vi "productsLow.vi"(8 "error in (no error)":errorcluster, 11 "reference in":refnum<class "Project Panels.lvclass">=refnum) -> (0 "error out":errorcluster, 3 "reference out":refnum<class "Project Panels.lvclass">)   [LabVIEW 2015, in "Project Panels.lvclass"]
uses:
  Project Panels.lvclass
  state.ctl
  <vilib>/Utility/miscctls.llb/LVRowAndColumnUnsignedTypeDef.ctl
  SYS/Devices Controller_llb/deviceType.ctl
  <vilib>/Utility/miscctls.llb/LVRowAndColumnTypeDef.ctl
  SYS/Devices Controller_llb/Devices Controller.lvclass
panel:
  out "title":string="Cosmed Asia Pacific - Products in Aussie"
  in  "tables":T1(tab)
  out "K5":string[][](table)=[["705001", "not active", "K4b2", "not active", "not active", "not active", "not active", "not active", "not active", "not active", "not active", "not active", ""], ["803033", "not active", "K4b2", "not active", "not active", "not active", "not active", "not active", "not active", "not active", "not active", "not active", ""], ["804042", "not active", "K4b2", "not active", "not active", "not active", "not active", "not active", "not active", "not active", "not active", "not active", ""], ["804046", "", "K4b2", "Univ. of Queensland", "St Lucia, Brisbane", "Gary Wilson", "seant@hms.uq.edu.au", "Bellamby", "sep-06", "Italy", "sep-07", "not active", ""], ["804047", "not active", "K4b2", "not active", "not active", "not active", "not active", "not active", "not active", "not active", "not active", "not active", ""], ["9806059", "6.2", "K4b2", "not active", "not active", "not active", "not active", "not active", "not active", "not active", "not active", "not active", ""], ["9806062", "5.1", "K4b2", "Queensland Academy of Sport", "Sunnybank", "Mark Andrews", "mark.andrews@srq.qld.com.au", "Nahtan, GC", "june 2013 in italy for CO2 refurbish", "Italy service", "jun-14", "", ""], ["9807077", "6.0a", "K4b2", "Uni of Canterbury", "Uni of Canterbury", "Gavin Blackwell", "gavin.blackwell@canterbury.ac.nz", "Christchurch", "feb-13", "fede", "feb-14", "", ""], ["9810080", "", "K4b2", "Royal Children's Hospital", "Herston", "Teresa Phillips", "Teresa_Phillips@health.qld.gov.au", "Herston", "jun-06", "Italy", "jun-07", "9/17/2013", ""], ["9903123", "7.2", "K4b2", "Uni of Adelaide", "Uni of Adelaide", "David Bentley", "david.bentley@adelaide.edu.au", "Adelaide", "dic-12", "Serv Italy +valve", "dic-13", "", ""], ["9912206", "7.3", "K4b2", "Uni of Canterbury", "Uni of Canterbury", "Gavin Blackwell", "gavin.blackwell@canterbury.ac.nz", "Christchurch", "feb-13", "fede", "feb-14", "", ""], ["200104325", "8", "K4b2", "Uni of South Australia", "Sansom Institute", "Michelle N. McDonnell", "", "Adelaide", "nov-11", "fede", "dic-12", "9/9/2013", ""], ["200201385", "9.1b", "K4b2", "University of Sydney", "Lidcombe Campus", "Hui Yin Ler  (PhD)", "", "Sydney", "oct-11", "fede", "oct-12", "9/9/2013", ""], ["200205419", "8.0", "K4b2", "University of Sydney", "Liverpool hospital", "Leanne Hassett", "leanne.hassett@sydney.edu.au", "Sydney", "nov-11", "fede", "nov-12", "Not Using in this moment", ""], ["200205423", "9.1b", "K4b2", "University of Sydney", "Lidcombe Campus", "Martin Thomson", "", "Sydney", "feb-10", "italy", "feb-11", "9/9/2013", ""], ["200205424", "7.3", "K4b2", "University of Sydney", "Lidcombe Campus", "Martin Thomson", "", "Sydney", "sep-08", "Italy", "sep-09", "9/10/2013", ""], ["200404607", "", "K4b2", "The Sydney Children's Hospital Network", "Westmead", "Leanne Purcell", "leanne.purcell@health.nsw.gov.au", "Westmead", "nov-08", "italy", "nov-09", "9/17/2013", "Yes, but waiting the start of the testing"], ["200512701", "8.0b", "K4b2", "James Cook Uni", "James Cook Uni", "Anthony Leight", "Anthony.Leicht@jcu.edu.au", "Townsville", "jan-13", "", "jan-14", "", ""], ["200601705", "", "K4b2", "Latrobe University", "Bundoora (Melb)", "Paul Moon", "P.Moon@latrobe.edu.au", "Melbourne", "jan-08", "Italy", "jan-09", "9/17/2013", ""], ["200607745", "", "K4b2", "QUT Brisbane", "Kelvin Grove", "Pei Cher", "pei.cher@qut.edu.au", "BBN", "may-13", "fede", "may-14", "", ""], ["200710813", "", "K4b2", "Victoria Uni", "", "Jessica Meilak", "jessica.meilak@vu.edu.au", "Melb", "jan-12", "Brad", "jan-14", "15/01/14", ""], ["200907909", "9.1b", "K4b2", "Uni of New South Wales", "Uni of New South Wales", "Stephen Redmond", "s.redmond@unsw.edu.au", "Sydney", "sep-12", "fede", "sep-13", "9/17/2013", ""], ["200909916", "", "K4b2", "Uni of Canterbury", "Uni of Canterbury", "Gavin Blackwell", "gavin.blackwell@canterbury.ac.nz", "Christchurch", "feb-13", "fede", "feb-14", "", ""], ["201007964", "", "K4b2", "University of Canberra", "Canberra", "Ben Rattray", "ben.rattray@canberra.edu.au", "Canberra", "mar-12", "", "mar-13", "9/17/2013", ""], ["201009980", "9.1b", "K4b2", "Uni of Technology Sydney", "UTS City Campus", "Steven Su", "steven.su@eng.uts.edu.au", "Sydney", "oct-12", "Medtel (also Lee Valve)", "oct-13", "9/17/2013", ""], ["2011121063", "", "K4b2", "Victoria Uni", "", "Jessica Meilak", "jessica.meilak@vu.edu.au", "Melb", "jan-12", "Brad", "jan-14", "", ""], ["2011121064", "", "K4b2", "Victoria Uni", "", "Jessica Meilak", "jessica.meilak@vu.edu.au", "Melb", "jan-12", "Brad", "jan-14", "", ""], ["2012021076", "", "K4b2", "Demo Unit", "Demo Unit", "TBD", "", "TBD", "sep-13", "Manu-AUS", "sep-14", "", ""], ["2012021080", "", "K4b2", "Massey Univ.", "Wellington", "Brandon Woolley", "B.Woolley@massey.ac.nz", "Wellington", "nov-13", "Manu-AUS", "nov-14", "", ""], ["2012061109", "", "K4b2", "Griffith University Gold Coast Campus", "Gold Coast", "Anna Boehm", "a.boehm@griffith.edu.au", "Gold Coast", "jul-13", "fede", "jul-14", "", ""], ["2012061115", "10.0d", "K4b2", "University of Newcastle", "Callaghan", "Robin Callister", "Robin.Callister@newcastle.edu.au", "Ourimbah", "nov-13", "Manu-AUS", "nov-14", "", ""], ["2012111144", "10.0d", "K4b2", "University of Newcastle", "Callaghan", "Robin Callister", "Robin.Callister@newcastle.edu.au", "Ourimbah", "nov-13", "Manu-AUS", "nov-14", "", ""], ["2012111148", "", "K4b2", "University of Western Sydney", "PENRITH", "Tara Hamilton", "t.hamilton@uws.edu.au", "PENRITH", "dec-13", "Manu-AUS", "dec-14", "", ""], ["2013011158", "10.0d", "K4b2", "University of the Sunshine Coast", "Maroochydore DC", "Ava Kerr", "akerr@usc.edu.au", "Sippy Downs", "may-13", "new", "may-14", "", ""], ["2013031168", "10.0d", "K4b2", "Australian Catholic University", "Sydney", "Phillip Chapman", "Phillip.Chapman@acu.edu.au", "Sydney", "apr-13", "new", "apr-14", "", ""], ["Prova", "", "Prova", "", "", "", "", "", "", "", "", "", ""]]
  out "k4b2":string[][](table)=[["705001", "not active", "K4b2", "not active", "not active", "not active", "not active", "not active", "not active", "not active", "not active", "not active", ""], ["803033", "not active", "K4b2", "not active", "not active", "not active", "not active", "not active", "not active", "not active", "not active", "not active", ""], ["804042", "not active", "K4b2", "not active", "not active", "not active", "not active", "not active", "not active", "not active", "not active", "not active", ""], ["804046", "", "K4b2", "Univ. of Queensland", "St Lucia, Brisbane", "Gary Wilson", "seant@hms.uq.edu.au", "Bellamby", "sep-06", "Italy", "sep-07", "not active", ""], ["804047", "not active", "K4b2", "not active", "not active", "not active", "not active", "not active", "not active", "not active", "not active", "not active", ""], ["9806059", "6.2", "K4b2", "not active", "not active", "not active", "not active", "not active", "not active", "not active", "not active", "not active", ""], ["9806062", "5.1", "K4b2", "Queensland Academy of Sport", "Sunnybank", "Mark Andrews", "mark.andrews@srq.qld.com.au", "Nahtan, GC", "june 2013 in italy for CO2 refurbish", "Italy service", "jun-14", "", ""], ["9807077", "6.0a", "K4b2", "Uni of Canterbury", "Uni of Canterbury", "Gavin Blackwell", "gavin.blackwell@canterbury.ac.nz", "Christchurch", "feb-13", "fede", "feb-14", "", ""], ["9810080", "", "K4b2", "Royal Children's Hospital", "Herston", "Teresa Phillips", "Teresa_Phillips@health.qld.gov.au", "Herston", "jun-06", "Italy", "jun-07", "9/17/2013", ""], ["9903123", "7.2", "K4b2", "Uni of Adelaide", "Uni of Adelaide", "David Bentley", "david.bentley@adelaide.edu.au", "Adelaide", "dic-12", "Serv Italy +valve", "dic-13", "", ""], ["9912206", "7.3", "K4b2", "Uni of Canterbury", "Uni of Canterbury", "Gavin Blackwell", "gavin.blackwell@canterbury.ac.nz", "Christchurch", "feb-13", "fede", "feb-14", "", ""], ["200104325", "8", "K4b2", "Uni of South Australia", "Sansom Institute", "Michelle N. McDonnell", "", "Adelaide", "nov-11", "fede", "dic-12", "9/9/2013", ""], ["200201385", "9.1b", "K4b2", "University of Sydney", "Lidcombe Campus", "Hui Yin Ler  (PhD)", "", "Sydney", "oct-11", "fede", "oct-12", "9/9/2013", ""], ["200205419", "8.0", "K4b2", "University of Sydney", "Liverpool hospital", "Leanne Hassett", "leanne.hassett@sydney.edu.au", "Sydney", "nov-11", "fede", "nov-12", "Not Using in this moment", ""], ["200205423", "9.1b", "K4b2", "University of Sydney", "Lidcombe Campus", "Martin Thomson", "", "Sydney", "feb-10", "italy", "feb-11", "9/9/2013", ""], ["200205424", "7.3", "K4b2", "University of Sydney", "Lidcombe Campus", "Martin Thomson", "", "Sydney", "sep-08", "Italy", "sep-09", "9/10/2013", ""], ["200404607", "", "K4b2", "The Sydney Children's Hospital Network", "Westmead", "Leanne Purcell", "leanne.purcell@health.nsw.gov.au", "Westmead", "nov-08", "italy", "nov-09", "9/17/2013", "Yes, but waiting the start of the testing"], ["200512701", "8.0b", "K4b2", "James Cook Uni", "James Cook Uni", "Anthony Leight", "Anthony.Leicht@jcu.edu.au", "Townsville", "jan-13", "", "jan-14", "", ""], ["200601705", "", "K4b2", "Latrobe University", "Bundoora (Melb)", "Paul Moon", "P.Moon@latrobe.edu.au", "Melbourne", "jan-08", "Italy", "jan-09", "9/17/2013", ""], ["200607745", "", "K4b2", "QUT Brisbane", "Kelvin Grove", "Pei Cher", "pei.cher@qut.edu.au", "BBN", "may-13", "fede", "may-14", "", ""], ["200710813", "", "K4b2", "Victoria Uni", "", "Jessica Meilak", "jessica.meilak@vu.edu.au", "Melb", "jan-12", "Brad", "jan-14", "15/01/14", ""], ["200907909", "9.1b", "K4b2", "Uni of New South Wales", "Uni of New South Wales", "Stephen Redmond", "s.redmond@unsw.edu.au", "Sydney", "sep-12", "fede", "sep-13", "9/17/2013", ""], ["200909916", "", "K4b2", "Uni of Canterbury", "Uni of Canterbury", "Gavin Blackwell", "gavin.blackwell@canterbury.ac.nz", "Christchurch", "feb-13", "fede", "feb-14", "", ""], ["201007964", "", "K4b2", "University of Canberra", "Canberra", "Ben Rattray", "ben.rattray@canberra.edu.au", "Canberra", "mar-12", "", "mar-13", "9/17/2013", ""], ["201009980", "9.1b", "K4b2", "Uni of Technology Sydney", "UTS City Campus", "Steven Su", "steven.su@eng.uts.edu.au", "Sydney", "oct-12", "Medtel (also Lee Valve)", "oct-13", "9/17/2013", ""], ["2011121063", "", "K4b2", "Victoria Uni", "", "Jessica Meilak", "jessica.meilak@vu.edu.au", "Melb", "jan-12", "Brad", "jan-14", "", ""], ["2011121064", "", "K4b2", "Victoria Uni", "", "Jessica Meilak", "jessica.meilak@vu.edu.au", "Melb", "jan-12", "Brad", "jan-14", "", ""], ["2012021076", "", "K4b2", "Demo Unit", "Demo Unit", "TBD", "", "TBD", "sep-13", "Manu-AUS", "sep-14", "", ""], ["2012021080", "", "K4b2", "Massey Univ.", "Wellington", "Brandon Woolley", "B.Woolley@massey.ac.nz", "Wellington", "nov-13", "Manu-AUS", "nov-14", "", ""], ["2012061109", "", "K4b2", "Griffith University Gold Coast Campus", "Gold Coast", "Anna Boehm", "a.boehm@griffith.edu.au", "Gold Coast", "jul-13", "fede", "jul-14", "", ""], ["2012061115", "10.0d", "K4b2", "University of Newcastle", "Callaghan", "Robin Callister", "Robin.Callister@newcastle.edu.au", "Ourimbah", "nov-13", "Manu-AUS", "nov-14", "", ""], ["2012111144", "10.0d", "K4b2", "University of Newcastle", "Callaghan", "Robin Callister", "Robin.Callister@newcastle.edu.au", "Ourimbah", "nov-13", "Manu-AUS", "nov-14", "", ""], ["2012111148", "", "K4b2", "University of Western Sydney", "PENRITH", "Tara Hamilton", "t.hamilton@uws.edu.au", "PENRITH", "dec-13", "Manu-AUS", "dec-14", "", ""], ["2013011158", "10.0d", "K4b2", "University of the Sunshine Coast", "Maroochydore DC", "Ava Kerr", "akerr@usc.edu.au", "Sippy Downs", "may-13", "new", "may-14", "", ""], ["2013031168", "10.0d", "K4b2", "Australian Catholic University", "Sydney", "Phillip Chapman", "Phillip.Chapman@acu.edu.au", "Sydney", "apr-13", "new", "apr-14", "", ""], ["Prova", "", "Prova", "", "", "", "", "", "", "", "", "", ""]]
  out "fitmate":string[][](table)=[["2005090013", "2.2", "Fitmate Pro", "Wesley Weight Management", "Milton", "Liz Ernst", "eernst@lifeshape.com.au", "Milton", "27/09", ""], ["2006020058", "1", "Fitmate WM", "Toombul Medical Centre", "Spring Hill", "Zoe Glover", "toombulmc@gmail.com", "Spring Hill", "27/09", ""], ["2006020059", "1", "Fitmate WM", "RMIT Univ.", "Melbourne", "George Lenon", "george.lenon@rmit.edu.au", "Melbourne", "27/09", ""], ["2006020060", "1", "Fitmate WM", "Logan Hospital", "Meadowbrook", "??", "??", "Meadowbrook", "", ""], ["2006020061", "1.6", "Fitmate WM", "Biomedex (Aust) Pty Ltd", "Woonona", "Biomedex (Aust) Pty Ltd", "??", "Woonona", "", ""], ["2006020077", "1", "Fitmate Pro", "Wesley Weight Management", "Southport", "Sally Jordan", "SJordan@weshealth.com.au", "Southport", "27/09 mail come back / no problem", ""], ["2006020078", "1", "Fitmate Pro", "Life4Ever Pty Ltd", "Arundel", "Michael Tait", "mail@drmichaeltait.com", "Arundel", "27/09 mail come back", ""], ["2006030062", "2.2", "Fitmate WM", "Biomedex (Aust) Pty Ltd", "Woonona", "Biomedex (Aust) Pty Ltd", "??", "Woonona", "", ""], ["2006030083", "2", "Fitmate Pro", "Australian College of Physical Education", "Olympic Park Sydney", "Sven Rees", "srees@acpe.edu.au", "Olympic Park Sydney", "30/09", ""], ["2006030084", "2.3", "Fitmate Pro", "Monash Univ. The Alfred Centre", "Frankston", "Tim Wallace", "tim.wallace@monash.edu", "Frankston", "Case Opned for Macro error", ""], ["2006030085", "2.2", "Fitmate Pro", "Southside Exercise Therapy", "Gymea", "Luke Delvecchio", "southsidepty@optusnet.com.au", "Gymea", "30/09", ""], ["2006060076", "1.1", "Fitmate WM", "Edith Cowan Univ.", "Joondalup", "Amanda Devine", "a.devine@ecu.edu.au", "Joondalup", "30/09", ""], ["2006060078", "1.1", "Fitmate WM", "Edith Cowan Univ.", "Joondalup", "Amanda Devine", "a.devine@ecu.edu.au", "Joondalup", "30/09", ""], ["2006060080", "2.3", "Fitmate WM", "WESLEY Corporate Health", "Brisbane", "Liz Ernst", "eernst@lifeshape.com.au", "Brisbane", "27/09", ""], ["2006080185", "1.1", "Fitmate Pro", "Edith Cowan Univ.", "Joondalup", "Doreen Mackie", "DMackie@hotmail.com", "Joondalup", "Waiting for details from email (n.vrdoljak@ecu.edu.au   )", ""], ["2006080186", "1.1", "Fitmate Pro", "Neocardia PTY LTD", "Noosaville", "Neavison", "Neavison@hotmail.com", "Noosaville", "30/09", ""], ["2006080187", "1.1", "Fitmate Pro", "Kams Health and Fitness", "Armidale", "Kamahl Barhoush", "info@kams.com.au", "Armidale", "doesn't answer/call again", ""], ["2006080188", "1.1", "Fitmate Pro", "Edith Cowan Univ.", "Joondalup", "Doreen Mackie", "DMackie@hotmail.com", "Joondalup", "Waiting for details from email (n.vrdoljak@ecu.edu.au   )", ""], ["2006080189", "1.1", "Fitmate Pro", "Get Back On Track", "Victoria", "Lisa Ham", "LisaH@bigpond.com.au", "Victoria", "doesn't answer/call again", ""], ["2006080190", "1.1", "Fitmate Pro", "Edith Cowan Univ.", "Joondalup", "Doreen Mackie", "DMackie@hotmail.com", "Joondalup", "Waiting for details from email (n.vrdoljak@ecu.edu.au   )", ""], ["2006080191", "1.1", "Fitmate Pro", "One Life", "PADDINGTON", "Justin Lang", "admin@onelifeliveit.net.au", "PADDINGTON", "01/10", "NOT ACTIVE"], ["2007030363", "1.1", "Fitmate Pro", "X-Fitness Systems Ltd", "Auckland,", "Scott Tibbutt", "scott@xfitness.co.nz", "Auckland,", "30/09", ""], ["2007030372", "1.1", "Fitmate Pro", "Edith Cowan Univ.", "Joondalup", "Doreen Mackie", "DMackie@hotmail.com", "Joondalup", "Waiting for details from email (n.vrdoljak@ecu.edu.au   )", ""], ["2007030373", "1.1", "Fitmate Pro", "Edith Cowan Univ.", "Joondalup", "Doreen Mackie", "DMackie@hotmail.com", "Joondalup", "Waiting for details from email (n.vrdoljak@ecu.edu.au   )", ""], ["2007030375", "1.1", "Fitmate Pro", "Vision Health and Fitness", "Toowoomba", "Troy Taylor", "troy@visionhealth.com.au", "Toowoomba", "30/09", ""], ["2007050155", "2", "Fitmate WM", "Fitness Fusion", "Ohope", "Erin Baker", "paul@fitnessfusion.co.nz", "Ohope", "30/09", ""], ["2007050156", "1.1", "Fitmate WM", "X-Fitness Systems Ltd", "Auckland,", "X-Fitness Systems Ltd", "jeremyu@uhl.co.nz", "Auckland,", "30/09", ""], ["2007050157", "2.2", "Fitmate WM", "Wesley Weight Management", "Milton", "Liz Ernst", "eernst@lifeshape.com.au", "Milton", "27/09", ""], ["2007050158", "2.2", "Fitmate WM", "WESLEY Corporate Health", "Brisbane", "Liz Ernst", "eernst@lifeshape.com.au", "Brisbane", "27/09", ""], ["2007050159", "1.1", "Fitmate WM", "Wesley Weight Management", "Rockhampton", "Simon Fawssett", "sfawssett@weshealth.com.au", "Rockhampton", "no problem", ""], ["2007050160", "2.2", "Fitmate WM", "WESLEY Corporate Health", "Brisbane", "Liz Ernst", "eernst@lifeshape.com.au", "Brisbane", "27/09", ""], ["2007050161", "1.1", "Fitmate WM", "Pyrmont Health & Fitness Club", "Pyrmont", "Antoine Poulter", "??", "Pyrmont", "", ""], ["2007050376", "1.1", "Fitmate Pro", "Edith Cowan Univ.", "Joondalup", "Doreen Mackie", "DMackie@hotmail.com", "Joondalup", "Waiting for details from email (n.vrdoljak@ecu.edu.au   )", ""], ["2007050377", "1.1", "Fitmate Pro", "Elgin Street Medical Centre", "Carlton", "Daniel Cobb", "dcobb@live.com.au", "Carlton", "30/09", ""], ["2007050378", "1.1", "Fitmate Pro", "Pyrmont Health & Fitness Club", "Pyrmont", "Justine Justine", "??", "Pyrmont", "", ""], ["2007050379", "1.6", "Fitmate Pro", "HERT", "Millers Point", "Mark Newton", "mark@hert.com.au", "Millers Point", "30/09", ""], ["2007050380", "1.1", "Fitmate Pro", "Edith Cowan Univ.", "Joondalup", "Doreen Mackie", "DMackie@hotmail.com", "Joondalup", "Waiting for details from email (n.vrdoljak@ecu.edu.au   )", ""], ["2007050381", "1.6", "Fitmate Pro", "Fitness Development Australia", "Sydney", "Fitness Development Australia", "zarko_mikulic@hotmail.com", "Sydney", "30/09", ""], ["2007050388", "1.1", "Fitmate Pro", "ULO Pty Ltd", "Roebourne Court", "Adam Brown", "adam@ulo.com.au", "Daisy Hill", "30/09", ""], ["2007050395", "1.6", "Fitmate Pro", "Biomedex (Aust) Pty Ltd", "Woonona", "Biomedex (Aust) Pty Ltd", "??", "Woonona", "", ""], ["2007050404", "1.1", "Fitmate Pro", "Biomedex (Aust) Pty Ltd", "Woonona", "Biomedex (Aust) Pty Ltd", "??", "Woonona", "", ""], ["2007060413", "2", "Fitmate Pro", "Biomedex (Aust) Pty Ltd", "Woonona", "Biomedex (Aust) Pty Ltd", "??", "Woonona", "", ""], ["2007060415", "1.1", "Fitmate Pro", "Mater Childrens Hospital", "South Brisbane", "Gary Leong", "gary.leong@mater.org.au", "South Brisbane", "1/10/2013", ""], ["2007060417", "1.1", "Fitmate Pro", "Ray Kelly Fitness", "Blacktown", "Ray Kelly", "maxvel01@hotmail.com", "Blacktown", "30/09", ""], ["2007100277", "2.2", "Fitmate WM", "Biomedex (Aust) Pty Ltd", "Woonona", "Biomedex (Aust) Pty Ltd", "??", "Woonona", "", ""], ["2007100278", "1.1", "Fitmate WM", "Tone Up Weight Loss", "Campbelltown", "Christopher Satara", "scott@swphysio.com.au'", "Campbelltown", "08/10", ""], ["2007100279", "1.6", "Fitmate WM", "Biomedex (Aust) Pty Ltd", "Woonona", "Biomedex (Aust) Pty Ltd", "??", "Woonona", "", ""], ["2007100281", "2.2", "Fitmate WM", "Biomedex (Aust) Pty Ltd", "Woonona", "Biomedex (Aust) Pty Ltd", "??", "Woonona", "", ""], ["2007100282", "2.2", "Fitmate WM", "Biomedex (Aust) Pty Ltd", "Woonona", "Biomedex (Aust) Pty Ltd", "??", "Woonona", "", ""], ["2007100484", "2.3", "Fitmate Pro", "Univ. of Auckland", "Auckland", "Grant Mawston", "", "Auckland", "", ""], ["2008010568", "2.3", "Fitmate Pro", "Australian College of", "Olympic Park Sydney", "Sven Rees", "srees@acpe.edu.au", "Olympic Park Sydney", "30/09", ""], ["2008010576", "2.2", "Fitmate Pro", "Body Dynamics Illawarra", "Bulli", "Alan Wilkie", "alan@bodydynamics.com.au", "Bulli", "01/10", ""], ["2008010578", "2.2", "Fitmate Pro", "Cardiofirst Pty Ltd.", "Frenchs Forest", "Camilla", "reports@cardiofirst.com.au", "Frenchs Forest", "", ""], ["2008010579", "2.2", "Fitmate Pro", "Biomedex (Aust) Pty Ltd", "Woonona", "Biomedex (Aust) Pty Ltd", "??", "Woonona", "", ""], ["2008010585", "1.1", "Fitmate Pro", "Biomedex (Aust) Pty Ltd", "Woonona", "Biomedex (Aust) Pty Ltd", "??", "Woonona", "", ""], ["2008030035", "1.6", "Fitmate MED", "Biomedex (Aust) Pty Ltd", "Woonona", "Biomedex (Aust) Pty Ltd", "??", "Woonona", "", ""], ["2008030037", "2", "Fitmate MED", "Biomedex (Aust) Pty Ltd", "Woonona", "Biomedex (Aust) Pty Ltd", "??", "Woonona", "", ""], ["2008040639", "1.5", "Fitmate Pro", "", "Wellington", "Stefan Darrall", "stefan.darrall@xtra.co.nz", "Wellington", "01/10", ""], ["2008040645", "2,2", "Fitmate Pro", "FEDERICO ZANELLA", "Narrabeen", "Federico Zanella", "", "Narrabeen", "", ""], ["2008090067", "2", "Fitmate MED", "Biomedex Pty Ltd.", "Bellambi", "Biomedex Pty Ltd.", "??", "Bellambi", "", ""], ["2008090071", "2", "Fitmate MED", "Logan City Council", "Logan Central", "Campbell MacGregor (not work there anymore)", "council@logan.qld.gov.au", "Logan Central", "08/10 request info sent", ""], ["2008090073", "1.6", "Fitmate MED", "Biomedex (Aust) Pty Ltd", "Woonona", "Biomedex (Aust) Pty Ltd", "??", "Woonona", "", ""], ["2008090075", "1.6", "Fitmate MED", "Enriched Health and Fizzsport Physiotherapy", "Port Macquarie", "Simon Turnball", "simon.turnbull@enrichedhealth.com.au", "Port Macquarie", "01/10", ""], ["2008090076", "2", "Fitmate MED", "Biomedex Pty Ltd.", "Bellambi", "Biomedex Pty Ltd.", "??", "Bellambi", "", ""], ["2008100402", "1.6", "Fitmate WM", "LSNDS P/L", "Mount Eliza", "Andrew Harland", "lsnds@optusenet.com.au", "Mount Eliza", "", ""], ["2008100403", "2.2", "Fitmate WM", "Monash Univ. The Alfred Centre", "Melbourne", "Emma Ridley", "emma.ridley@monash.edu", "Melbourne", "01/10", ""], ["2008100404", "1.6", "Fitmate WM", "The Prince Charles Hospital", "Brisbane", "Renee Rogers", "", "Brisbane", "", ""], ["2008100405", "2.2", "Fitmate WM", "Monash Univ. The Alfred Centre", "Melbourne", "Emma Ridley", "emma.ridley@monash.edu", "Melbourne", "01/10", ""], ["2008100408", "1.6", "Fitmate WM", "Univ. of Newcastle (AUSTRALIA)", "Tamworth", "Leanne Brown", "leanne.brown@newcastle.edu.au", "Tamworth", "01/10", ""], ["2009070009", "1,6", "Fitmate Pro", "Ray Kelly Fitness", "Blacktown", "Ray Kelly", "maxvel01@hotmail.com", "Blacktown", "30/09", ""], ["2010011057", "2", "Fitmate Pro", "Swift Sports Performance Equip", "Lismore", "Mark Fisher", "mark@spe.com.au", "Lismore", "01/10", ""], ["2010021097", "2", "Fitmate Pro", "ASCENCIA Pty. Limited", "Notting Hill", "Michael Panagopoulos", "michael@ascencia.com.au", "Notting Hill", "", ""], ["2010021098", "2", "Fitmate Pro", "Melbourne Sports & Allied Health Clinic", "Essendon North", "Simon Sostaric", "simon@msahc.com.au", "Essendon North", "01/10", ""], ["2010041123", "2", "Fitmate Pro", "Pymble Ladies College", "Pymble", "Thomas Kindred", "tkindred@pymblelc.nsw.edu.au", "Pymble", "01/10", ""], ["2010041133", "2", "Fitmate Pro", "New Zealand Institute of Sport", "Wellington", "Tony Rogers", "tony.r@nzis.co.nz", "Wellington", "info da fede", ""], ["2010091200", "2", "Fitmate Pro", "Univ. of Western Sydney", "Sydney", "Andrew Webber", "a.webber@uws.edu.au / a.boros@uws.edu.au", "Sydney", "01/10", ""], ["2010091208", "2.2", "Fitmate Pro", "AusFitness Test", "Burleigh Heads", "Daniel Mckenzie", "dan@ausfitnesstest.com", "Burleigh Heads", "01/10", ""], ["2010111079", "2", "Fitmate MED", "Xceler8", "Wagga", "Kerry Podmore", "Kerry-xceler8@bigpond.com", "Wagga", "01/10", ""], ["2010121080", "2", "Fitmate MED", "", "Toormina, Boambee", "Chris Cherry", "", "Toormina, Boambee", "", ""], ["2010121084", "2", "Fitmate MED", "Victoria University", "St.ALbans", "Christos Stathis", "christos.stathis@vu.edu.au", "St.ALbans", "01/10", ""], ["2010121085", "2", "Fitmate MED", "Victoria University", "St.ALbans", "Christos Stathis", "christos.stathis@vu.edu.au", "St.ALbans", "01/10", ""], ["2010121088", "2", "Fitmate MED", "", "Melbourne Nth.", "T. Goh", "??", "Melbourne Nth.", "", ""], ["2010121250", "2.2", "Fitmate Pro", "Otago Polytechnic", "Dunedin", "Hayden Croft", "Hayden.Croft@op.ac.nz", "Dunedin", "01/10", ""], ["2011021095", "2", "Fitmate MED", "CHM Management", "South Melbourne", "Kirsty Lerm", "klerm@chm.com.au", "South Melbourne", "01/10", ""], ["2011041238", "2.2", "Fitmate WM", "University of the Sunshine Coast", "Sippy Downs", "Gary Slater", "gslater@usc.edu.au", "Maroochydore DC", "01/10", "accepted 04/10"], ["2011061360", "2.2", "Fitmate Pro", "Sports Orthopaedic and Rehabilitation", "Sydney", "Peter McDonald", "pmcdfitness@gmail.com.au'", "Sydney", "", ""], ["2011061363", "2.2", "Fitmate Pro", "Sports Orthopaedic and Rehabilitation", "Sydney", "Peter McDonald", "pmcdfitness@gmail.com.au'", "Sydney", "", ""], ["2011071270", "2.2", "Fitmate WM", "University of Otago", "Dunedin", "Gavin Hendry", "gavin.hendry@otago.ac.nz", "Dunedin", "01/10", ""], ["2011111148", "2", "Fitmate MED", "JLM Accutek Health", "Homebush", "Lorrence(Lorenzo) Platania", "??", "Homebush", "", ""], ["2011111155", "2", "Fitmate MED", "JLM Accutek Health", "Homebush", "Lorrence(Lorenzo) Platania", "??", "Homebush", "", ""], ["2011121441", "2.2", "Fitmate Pro", "The Scots College", "Bellevue Hill", "Tenzing Tsewang", "t.tsewang@tsc.nsw.edu.au", "Bellevue Hill", "01/10", ""], ["2011121443", "2.2", "Fitmate Pro", "Sydney Sports & Exercise", "Sydney Olympic Park", "Dean McNamara", "", "Sydney Olympic Park", "", ""], ["2012031327", "2.2", "Fitmate WM", "Univ. of Adelaide", "Adelaide", "Univ. of Adelaide", "", "Adelaide", "", ""], ["2012050009", "2,3", "Fitmate GS", "Belconnen Specialist Center", "Bruce-Canberra", "Mariame Iraki", "", "Bruce-Canberra", "", ""], ["2012061551", "2.2", "Fitmate Pro", "The Scots College", "Bellevue Hill", "Tenzing Tsewang", "t.tsewang@tsc.nsw.edu.au", "Bellevue Hill", "01/10", ""], ["2012061552", "2.2", "Fitmate Pro", "The Scots College", "Bellevue Hill", "Tenzing Tsewang", "t.tsewang@tsc.nsw.edu.au", "Bellevue Hill", "01/10", ""], ["2012061554", "2.2", "Fitmate Pro", "The Scots College", "Bellevue Hill", "Tenzing Tsewang", "t.tsewang@tsc.nsw.edu.au", "Bellevue Hill", "01/10", ""], ["2012091028", "2,3", "Fitmate GS", "The University of Newcastle (AUS)", "Callaghan", "Anna Bukey", "Anna.Bukey@newcastle.edu.au", "Callaghan", "01/10", ""], ["2012101617", "2.3", "Fitmate Pro", "FEDERICO ZANELLA", "Narrabeen", "Federico Zanella", "", "Narrabeen", "", ""], ["2012101619", "2.3", "Fitmate Pro", "Adelaide Exercise Physiology (AEP)", "", "Reuben Vanderzalm", "reuben@aep.net.au", "", "01/10", ""], ["2012111654", "2.2", "Fitmate Pro", "Vascular Ultrasound Partners Pty Ltd", "Adelaide", "Jim Gotting", "emac2403@gmail.com", "Adelaide", "01/10", ""], ["2013011031", "2,3", "Fitmate GS", "FEDERICO ZANELLA", "Narrabeen", "Federico Zanella", "", "Narrabeen", "", ""], ["2013021388", "2.2", "Fitmate WM", "Monash Univ. The Alfred Centre", "Melbourne", "Emma Ridley", "emma.ridley@monash.edu", "Melbourne", "01/10", ""], ["2013041734", "2.2", "Fitmate Pro", "SA Ambulance", "Eastwood", "Adam Zerner", "adam.zerner@health.sa.gov.au", "Eastwood", "01/10", ""], ["2013061753", "2.2", "Fitmate Pro", "James Cook University", "Douglas", "Anthony Leight", "Anthony.Leicht@jcu.edu.au", "Townsville", "01/10", ""], ["20050800003", "1.6", "Fitmate Pro", "Biomedex (Aust) Pty Ltd", "Woonona", "Biomedex (Aust) Pty Ltd", "??", "Woonona", "", ""]]
  out "RMR":string[][](table)=[["2009010042", "", "RMR + ICU", "Monash Univ. The Alfred Centre", "Melbourne", "Emma Ridley", "Emma.Ridley@med.monash.edu.au", "Melbourne", "", ""], ["2010020172", "", "RMR + ICU", "Prince Charles Hospital", "Brisbane", "Vanessa King", "Vanessa_King@health.qld.gov.au", "Brisbane", "", ""], ["2010080174", "", "RMR + ICU", "Monash Univ. The Alfred Centre", "Melbourne", "Emma Ridley", "Emma.Ridley@med.monash.edu.au", "Melbourne", "", ""], ["2010110180", "", "RMR + ICU", "Monash Univ. The Alfred Centre", "Melbourne", "Emma Ridley", "Emma.Ridley@med.monash.edu.au", "Melbourne", "", ""], ["2010110181", "", "RMR + ICU", "Gold Coast Hospital and Robina", "Southport", "Alan Spencer", "alan_spencer@healthqld.gov.au", "Southport", "", ""], ["2011050212", "", "RMR + ICU", "John Hunter Hospital", "New Lambton Heights", "Justin Singleton", "justin.singleton@hnehealth.nsw.gov.au", "New Lambton Heights", "", ""], ["2011110238", "", "RMR", "Royal Prince Alfred Hospital", "Camperdown", "Joanne Heyman", "joanne.heyman@sswahs.nsw.gov.au", "Camperdown", "", ""], ["2012110294", "", "RMR", "University of the Sunshine Coast", "Maroochydore DC", "Gary Slater", "gslater@usc.edu.au", "Maroochydore DC", "", ""], ["2013020316", "", "RMR + ICU", "Royal Perth Hospital", "Perth", "Wayne Epton", "wayne.epton@health.wa.gov.au", "Perth", "", ""], ["2013050335", "", "RMR + ICU", "Gold Coast Hospital and Robina", "Southport", "Alan Spencer", "alan_spencer@healthqld.gov.au", "Southport", "", ""], ["2013050332", "", "RMR", "Auckland City Hospital", "Auckland", "Shay McGuinness", "", "Auckland", "", ""], ["2013050330", "", "RMR + ICU", "University of Queensland", "Herston", "Alexia Murphy", "alexia.murphy@uq.edu.au", "Herston", "", ""]]
  out "CPET":string[][](table)=[["9807035", "5", "Quark b2", "The Royal Melbourne Institute of Technology - RMIT", "Bundoora", "", "", "", "", ""], ["9901046", "", "Quark b2", "Biomedex", "", "", "", "", "", ""], ["9905053", "5.1a", "Quark b2", "Baker Medical Research Institute", "", "", "", "", "", ""], ["200601281", "", "Quark b2", "Ultra Thoroughbred Racing Pty. Ltb", "Green Iris", "Rod Cedaro", "rod.cedaro@gmail.com", "Rod Cedaro", "", ""], ["2007060003", "", "Quark CPET", "Liverpool Hospital", "Liverpool", "Mark Newman", "Mark.Newman@sswahs.nsw.gov.au", "Liverpool", "", ""], ["2008030037", "10.0d", "Quark CPET", "University Otago", "Dunedin", "Nigel Barrett", "nigel.barrett@otago.ac.nz", "Dunedin", "", ""], ["2008030006", "", "Quark PFT/CPET Nutritional", "University Otago", "Dunedin", "Dene Irvine", "dene.irvine@otago.ac.nz", "Dunedin", "", ""], ["2008050039", "9", "Quark CPET", "Victorian Institute of Sport", "Melbourne", "Simon Blundell", "simon.blundell@vis.org.au", "Melbourne", "", ""], ["2008120093", "9.1b", "Quark CPET", "Griffith University Gold Coast Campus", "Gold Coast", "Caroline Young", "caroline.b.young@griffith.edu.au", "Gold Coast", "", ""], ["2009100185", "10.0d", "Quark CPET", "University of Otago", "Dunedin", "Nigel Barrett", "nigel.barrett@otago.ac.nz", "Dunedin", "", ""], ["2010020214", "", "Quark CPET", "Canberra Hospital", "Garran", "Leonard Arnolda", "", "Garran", "", ""], ["2011110397", "10.0d", "Quark CPET", "Univ. of Sydney", "Lidcombe", "Corinne Caillaud", "corinnecalillaud@sidney.edu.au", "Lidcombe", "", ""], ["2011110398", "10.0d", "Quark CPET", "Univ. of Sydney", "Lidcombe", "Corinne Caillaud", "corinnecalillaud@sidney.edu.au", "Lidcombe", "", ""], ["2012020412", "10.0d", "Quark CPET", "University of Otago", "Dunedin", "Nigel Barrett", "nigel.barrett@otago.ac.nz", "Dunedin", "", ""], ["2011120402", "10.0d", "Quark CPET", "The Scots College", "Bellevue Hill", "Tenzing Tsewang", "t.tsewang@tsc.nsw.edu.au", "Bellevue Hill", "", ""], ["2012100477", "10.0d", "Quark CPET", "Victoria University", "Footscray", "Jessica Meilak", "jessica.meilak@vu.edu.au", "Footscray", "", ""], ["2012060085", "10.0d", "Quark CPET", "Victoria University", "Melbourne", "Bradley Gatt", "bradley.gatt@vu.edu.au", "Melbourne", "", ""], ["2012120094", "10.0e", "Quark CPET", "Fede", "DEMO", "DEMO", "DEMO", "DEMO", "", ""], ["2013020524", "", "Quark CPET", "Australian Catholic University - ACU", "Strathfield", "Anoj Poudyal", "anoj.poudyal@acu.edu.au", "Strathfield", "", ""], ["2013060561", "", "Quark CPET", "James Cook University", "Townsville", "Anthony Leight", "Anthony.Leicht@jcu.edu.au", "Douglas", "", ""], ["2013110612", "", "Quark CPET", "Australian Catholic University BBN", "Virginia", "Tim Blackmore", "tim.blackmore@acu.edu.au", "Banyo", "", ""], ["2013120110", "", "Quark CPET", "Australian Catholic University BBN", "Virginia", "Tim Blackmore", "tim.blackmore@acu.edu.au", "Banyo", "", ""]]
  out "BB-PFT":string[][](table)=[["2009010042", "", "RMR + ICU", "Monash Univ. The Alfred Centre", "Melbourne", "Emma Ridley", "Emma.Ridley@med.monash.edu.au", "Melbourne", "", ""], ["2010020172", "", "RMR + ICU", "Prince Charles Hospital", "Brisbane", "Vanessa King", "Vanessa_King@health.qld.gov.au", "Brisbane", "", ""], ["2010080174", "", "RMR + ICU", "Monash Univ. The Alfred Centre", "Melbourne", "Emma Ridley", "Emma.Ridley@med.monash.edu.au", "Melbourne", "", ""], ["2010110180", "", "RMR + ICU", "Monash Univ. The Alfred Centre", "Melbourne", "Emma Ridley", "Emma.Ridley@med.monash.edu.au", "Melbourne", "", ""], ["2010110181", "", "RMR + ICU", "Gold Coast Hospital and Robina", "Southport", "Alan Spencer", "alan_spencer@healthqld.gov.au", "Southport", "", ""], ["2011050212", "", "RMR + ICU", "John Hunter Hospital", "New Lambton Heights", "Justin Singleton", "justin.singleton@hnehealth.nsw.gov.au", "New Lambton Heights", "", ""], ["2011110238", "", "RMR", "Royal Prince Alfred Hospital", "Camperdown", "Joanne Heyman", "joanne.heyman@sswahs.nsw.gov.au", "Camperdown", "", ""], ["2012110294", "", "RMR", "University of the Sunshine Coast", "Maroochydore DC", "Gary Slater", "gslater@usc.edu.au", "Maroochydore DC", "", ""], ["2013020316", "", "RMR + ICU", "Royal Perth Hospital", "Perth", "Wayne Epton", "wayne.epton@health.wa.gov.au", "Perth", "", ""], ["2013050335", "", "RMR + ICU", "Gold Coast Hospital and Robina", "Southport", "Alan Spencer", "alan_spencer@healthqld.gov.au", "Southport", "", ""], ["2013050332", "", "RMR", "Auckland City Hospital", "Auckland", "Shay McGuinness", "", "Auckland", "", ""], ["2013050330", "", "RMR + ICU", "University of Queensland", "Herston", "Alexia Murphy", "alexia.murphy@uq.edu.au", "Herston", "", ""]]
  out "BP":string[][](table)=[["1018", "", "BP GS", "Uni of Adelaide", "Adelaide", "", "", "", "", ""], ["3054", "", "BP DOS", "Uni of Queensland", "Brisbane", "", "", "", "", ""], ["3268", "", "BP DOS W", "Queensland Univ. of Technology", "Kelvin grove", "Rachel Wood", "re.wood@qut.edu.au", "Kelvin grove", "", ""], ["3367", "", "BP W", "Queensland University of Technology", "Kelvin Grove", "Rachel Wood", "re.wood@qut.edu.au", "", "", ""], ["3436", "", "BP W", "Princess Margaret Hospital for Children", "Perth", "David Forbes", "david.forbes@health.wa.gov.au", "Perth", "", ""], ["3529", "5.1.0", "BP GS", "Monash Medical Centre", "Clayton", "Sharon Marks", "sharon@fpds.com.au", "Clayton", "", ""], ["3562", "", "BP GS", "Massey University", "Palmerston North", "Kevin Pedley", "k.c.pedley@massey.ac.nz", "Palmerston North", "", ""], ["3563", "4.2.4", "BP GS", "Bodyology Exercise Science Studio", "Notting Hill", "Andrew Garlick", "andrew@bodyologystudio.com.au", "Notting Hill", "", ""], ["3640", "", "BP GS", "Wesley Research Institute", "Toowong", "Greg Hafner", "ghafner@wesleyresearch.com.au", "Toowong", "", ""], ["3788", "", "BP GS", "Federico", "Federico", "Federico", "", "Federico", "", ""], ["3793", "", "BP GS", "University of the Sunshine Coast", "Maroochydore DC", "Gary Slater", "gslater@usc.edu.au", "Maroochydore DC", "", ""], ["3821", "", "BP GS", "The Scots College", "Bellevue Hill", "Tenzing Tsewang", "t.tsewang@tsc.nsw.edu.au", "Bellevue Hill", "", ""], ["3852", "", "BP GS", "Univ. of Adelaide", "Adelaide", "Univ. of Adelaide", "", "Adelaide", "", ""], ["3868", "5.2.0", "BP GS", "Univ. of Sydney", "Sydney", "Amanda Sainsbury Salis", "amanda.sainsbury-salis@sydney.edu.au", "Sydney", "", ""], ["3930", "", "BP GS", "Paula Serena Pool", "Townsville", "Paula Serena Pool", "", "Townsville", "", ""], ["3947", "", "BP GS", "Paula Serena Pool", "Townsville", "Paula Pool", "", "West End", "", ""], ["3993", "", "BP GS", "Queensland Univ. of Technology", "Kelvin grove", "Nuala Byrne", "n.byrne@qut.edu.au", "Kelvin grove", "", ""], ["4063", "", "BP ST", "Queensland Univ. of Technology", "Kelvin grove", "Rachel Wood", "re.wood@qut.edu.au", "Kelvin grove", "", ""], ["4539", "", "BP EX", "World Gym Ashmore", "Ashmore", "Sarah Friebe", "sarah@worldgymashmore.com.au", "Ashmore", "", ""], ["COSEMD USA 1", "", "BP GS", "University of the Sunshine Coast", "Maroochydore DC Qld", "University of the Sunshine Coast", "", "Maroochydore DC Qld", "", ""]]
  out "PP":string[][](table)=[["6025", "", "PP", "King Edward Memorial", "Perth", "Gemma McLeod", "mcleod.gemma1@gmail.com", "Perth", "", ""], ["6088", "", "PP", "Univ. of Sydney", "Penrith", "Ralph Nanan", "ralph.nanan@sydney.edu.au", "Penrith", "", ""], ["6021", "", "PP", "University of Queensland Centre for Clinical Research", "Herston", "Barbara Lingwood", "b.lingwood@uq.edu.au", "Herston", "", ""], ["6023", "", "PP", "University of Queensland Centre for Clinical Research", "Herston", "Barbara Lingwood", "b.lingwood@uq.edu.au", "Herston", "", ""], ["6082", "", "PP", "Massey Univ.", "Palmerston North", "Jane Coad", "CoadJ.Coad@massey.ac.nz", "Palmerston North", "", ""], ["6044", "", "PP", "Royal Prince Alfred Hospital", "Camperdown", "Emily Bek", "emily.bek@sydney.edu.au", "Camperdown", "", ""]]
  in  "Delete Item":bool
  in  "Send Follow Up":bool
  in  "Search Item":bool
  in  "Edit Item":bool
  in  "New Item":bool
  out "Item Selected (S/N):":string
  out "statuBar":string
  in  "Stop Button":bool
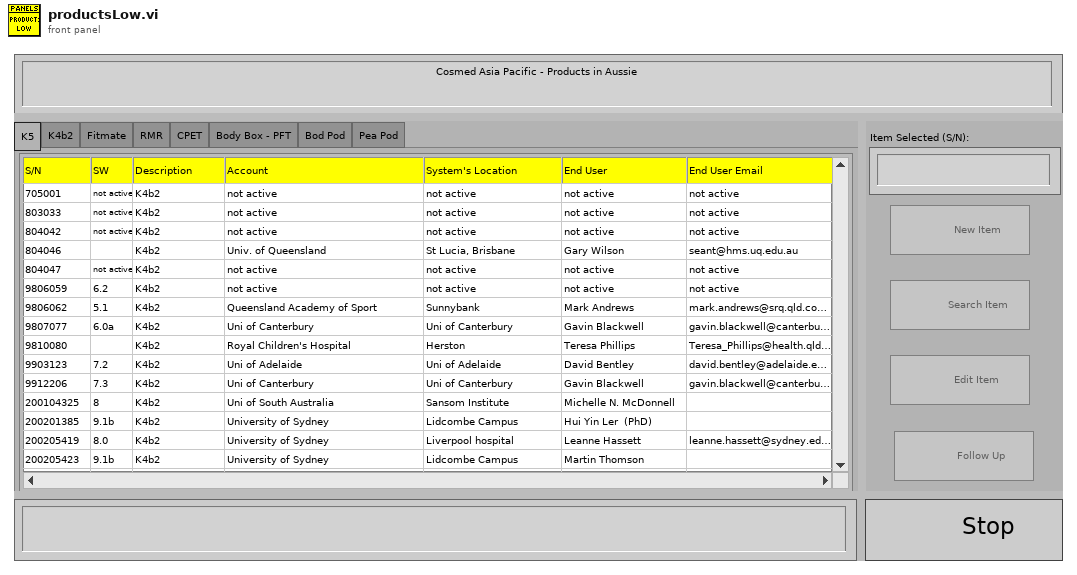
[diagram p1: front panel]
types:
  T1 = enum32{"K5", "K4b2", "Fitmate", "RMR", "CPET", "Body Box - PFT", "Bod Pod", "Pea Pod"}
  T2 = typedef "Project Panels.lvclass/state.ctl" = enum16{"initiate", "waitEvent", "newItem", "searchItem", "editItem", "sendFollowUp", "deleteItem", "save", "stop"}
  T3 = typedef "LVRowAndColumnUnsignedTypeDef.ctl" = cluster{"Row":u32, "Column":u32}
  T4 = enum8{"Enabled", "Disabled", "Disabled and Grayed Out"}
  T5 = typedef "Devices Controller.lvclass/deviceType.ctl" = enum16{"k5", "k4b2", "fitmate", "cpet", "rmr", "bodyBoxPft", "bp", "pp"}
  T6 = typedef "LVRowAndColumnTypeDef.ctl" = cluster{"Row":i32, "Column":i32}
  T7 = typedef "Project Panels.lvclass/ObjectAttributesRef.ctl" = refnum<data-value>
  T8 = typedef "Project Panels.lvclass/ObjectAttributes.ctl" = cluster{"MyAttribute":dbl, "device_controller_ref":refnum<class "Devices Controller.lvclass">, "file_controller_ref":refnum<class "File Controller.lvclass">, "item_controller_ref":refnum<class "Items Controller.lvclass">, "item_tables":cluster{"checkIN":string[][], "checkOUT":string[][], "storage":string[][]}, "quickbook_table":cluster{"notes":string[][]}, "notification_controller_ref":refnum<class "Notification Controller.lvclass">, "partstracking_controller_ref":refnum<class "PartsTracking Controller.lvclass">, "product_tables":cluster{"k4b2":string[][], "fitmate":string[][], "RMR":string[][], "CPET":string[][], "BP":string[][], "PP":string[][], "k5":string[][], "bb-pft":string[][]}, "rowsColour":u32[], "low_resolution?":bool, "run_python?":bool}
  T9 = cluster{"k4b2":string[][], "fitmate":string[][], "RMR":string[][], "CPET":string[][], "BP":string[][], "PP":string[][], "k5":string[][], "bb-pft":string[][]}
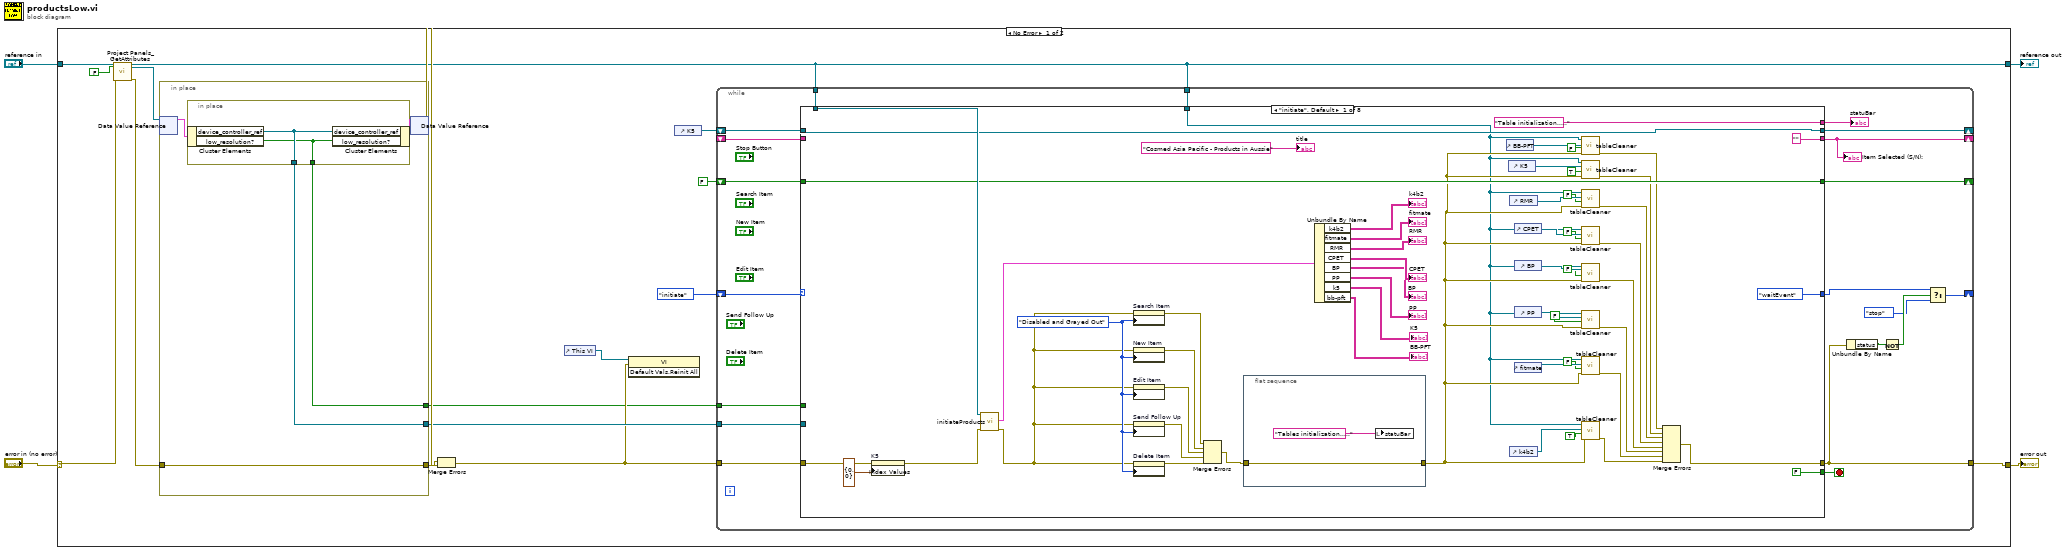
[diagram p0: block diagram]
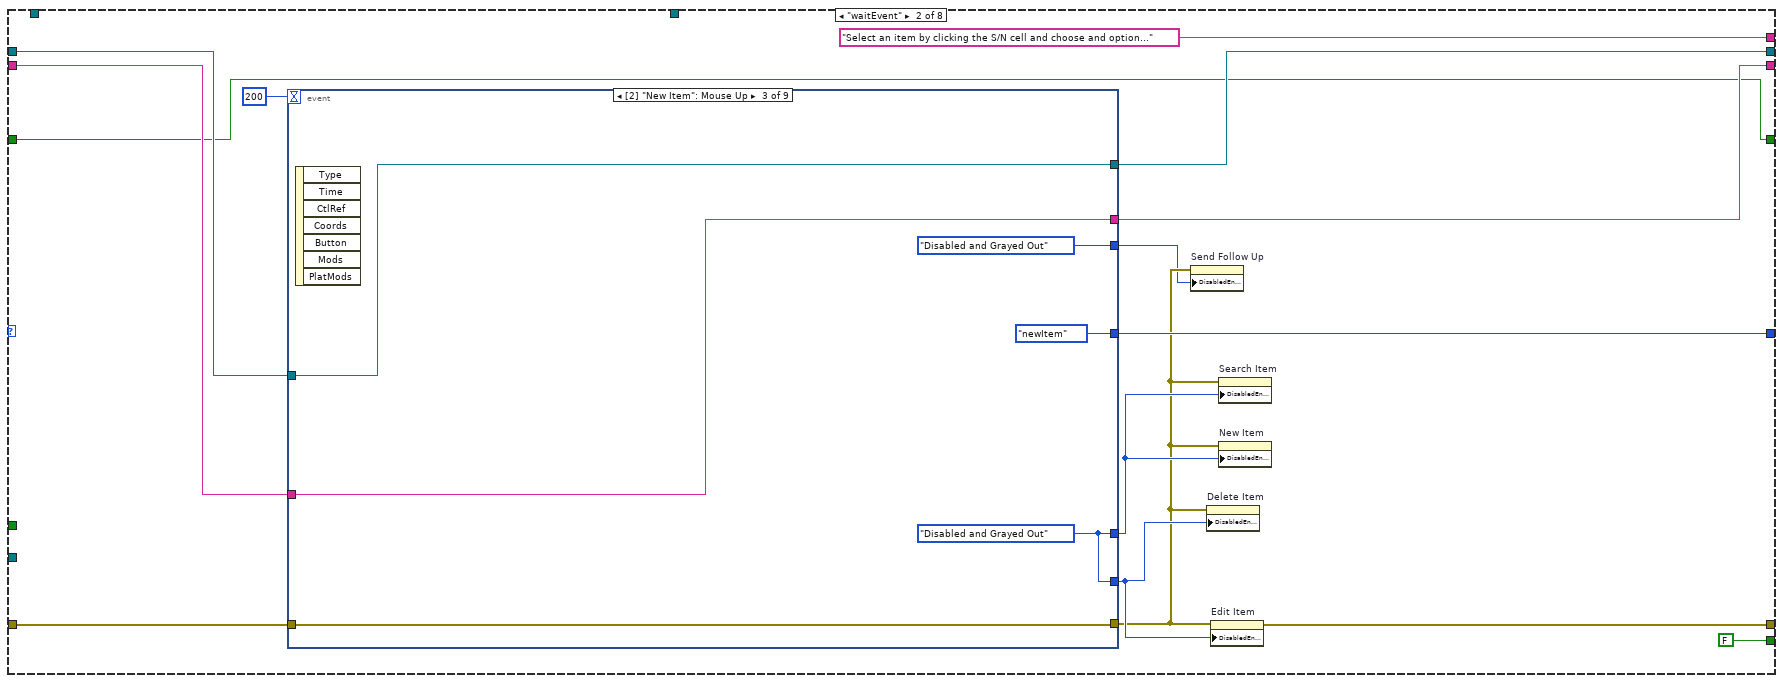
[diagram p2: hidden frame]
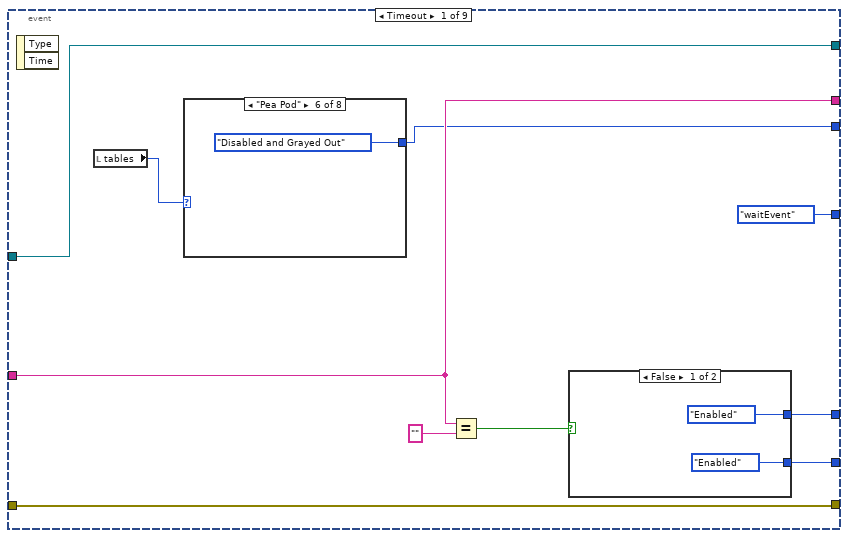
[diagram p3: hidden frame]
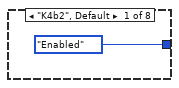
[diagram p4: hidden frame]
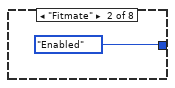
[diagram p5: hidden frame]
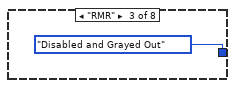
[diagram p6: hidden frame]
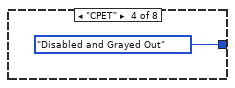
[diagram p7: hidden frame]
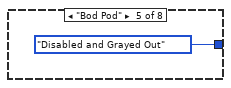
[diagram p8: hidden frame]
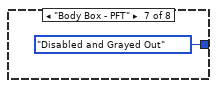
[diagram p9: hidden frame]
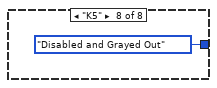
[diagram p10: hidden frame]
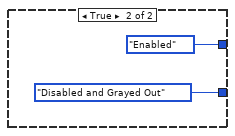
[diagram p11: hidden frame]
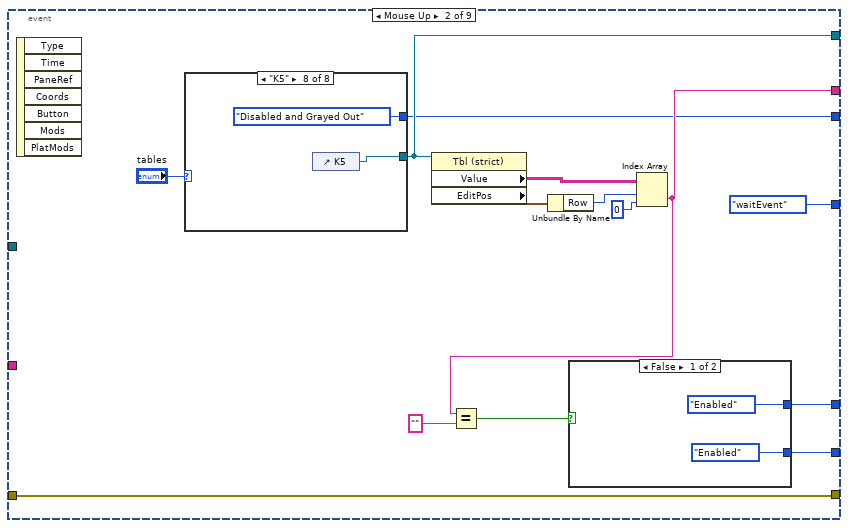
[diagram p12: hidden frame]
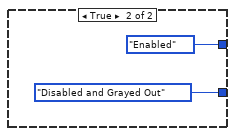
[diagram p13: hidden frame]
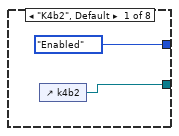
[diagram p14: hidden frame]
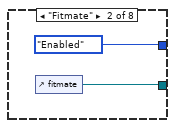
[diagram p15: hidden frame]
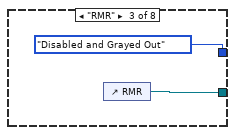
[diagram p16: hidden frame]
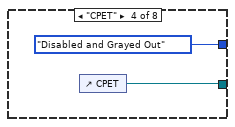
[diagram p17: hidden frame]
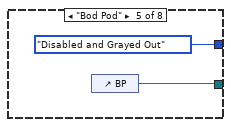
[diagram p18: hidden frame]
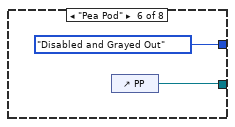
[diagram p19: hidden frame]
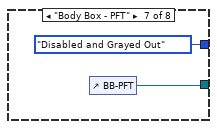
[diagram p20: hidden frame]
diagram:
  n1 = case shown="No Error" "error in (no error)" {
    selector: "error in (no error)" -> [w16 w423]
    tunnel: [w13 w423] -> w3
    tunnel: [w11 w422] -> w1
    tunnel: "reference in" -> [w18 w422]
    frame No Error {
      n2 = call "Project Panels_GetAttributes.vi"("reference in"=w18, "return data? (T)"=FALSE, "error in (no error)"=w16) -> ("reference out"=w11:refnum<class "Project Panels.lvclass">, "attributes ref"=w14:T7, "error out"=w15:errorcluster)  [unwired: 13 in, 1 out]
      n3 = in-place {
        in-place-border: w15 -> [w417]
        in-place-border: [w417] -> w19
        in-place-border: [w416] -> w7
        in-place-border: [w415] -> w5
        n4 = in-place-dvr #1(w14) -> (w418:T8)  [unwired: 1 out]
        n5 = in-place {
          in-place-border: [w421] -> w416
          in-place-border: [w420] -> w415
          n6 = in-place-cluster #2(w418) -> ("device_controller_ref"=w421:refnum<class "Devices Controller.lvclass">, "low_resolution?"=w420:bool)
          n7 = in-place-cluster #2("device_controller_ref"=w421, "low_resolution?"=w420) -> (w419:T8)
        }
        n8 = in-place-dvr #1(w419) -> (w20:errorcluster)  [unwired: 1 out]
      }
      n9 = Merge Errors(w19, w20) -> (w6:errorcluster)
      n10 = control-ref of="This VI"() -> (w9:refnum<vi>)
      n11 = invoke class="VI" method="Default Vals.Reinit All"(reference=w9, error in=w6) -> ()  [unwired: 1 in, 3 out]
      n12 = control-ref of="K5"() -> (w10:refnum<vi>)
      n13 = while {
        tunnel: w11 -> [w40]
        tunnel: w6 -> [w39]
        tunnel: [w37] -> w13
        shift-right: [w34] -> _
        shift-left: state."initiate" ("state") -> [w38]
        shift-right: [w29] -> _
        shift-left: _ -> [w28]
        shift-right: [w27] -> _
        shift-left: w10 -> [w26]
        tunnel: w11 -> [w25]
        shift-right: [w24] -> _
        shift-left: FALSE ("saved?") -> [w23]
        tunnel: w7 -> [w22]
        tunnel: w5 -> [w21]
        stop <- w31 stop-if-true
        n14 = case shown="\"initiate\", Default" w38 {
          tunnel: w40 -> [w47 _ w229 w263 w293 w323 w366 _]
          tunnel: w39 -> [w43 w111 w231 w262 w291 w326 w365 w393]
          tunnel: [w44 w102 w227 w261 w276 w318 w367 w392] -> w37
          tunnel: [state."waitEvent" ("state") w109 w224 w258 w275 w321 w359 state."stop" ("state")] -> w35
          tunnel: [FALSE FALSE FALSE FALSE FALSE FALSE FALSE TRUE] -> w31
          tunnel: ["Table initialization....." ("title") "Select an item by clicking the S/N cell and choose and option..." ("title") "New Item option selected...." ("title") "Search Item option selected..." ("title") "Edit Item option selected..." ("title") "Send Follow Up option selected" ("title") "Delete Item option selected..." ("title") w398] -> w30
          tunnel: ["" w101 "" "" w284 w322 w362 w401] -> w29
          tunnel: w28 -> [_ w107 _ _ w284 w322 w362 w401]
          tunnel: [w57 w100 w232 w264 w288 w325 w363 w397] -> w27
          tunnel: w26 -> [w57 w103 w232 w264 w288 w325 w363 w397]
          tunnel: w25 -> [w58 _ _ _ _ _ _ _]
          tunnel: [w55 w98 w223 w256 w271 w320 w357 FALSE ("saved?")] -> w24
          tunnel: w23 -> [w55 w98 w220 w254 w269 w320 w355 w391]
          tunnel: w22 -> [_ _ _ _ _ _ _ w390]
          tunnel: w21 -> [_ _ w218 _ w268 _ w352 _]
          frame "initiate", Default {
            w60 = T4."Disabled and Grayed Out" ("Disabled")
            n15 = property on="K5" class="Tbl (strict)"(error in=w43, "Index Values"=T3 {"Row"=0, "Column"=0}) -> (error out=w42:errorcluster)  [unwired: 1 in, 1 out]
            n16 = call "initiateProducts.vi"("reference in"=w58, "error in (no error)"=w42) -> ("tables"=w56:T9, "error out"=w59:errorcluster)  [unwired: 15 in, 1 out]
            n17 = property on="Search Item" class="Bool"(error in=w59, "DisabledEnum"=w60) -> (error out=w61:errorcluster)  [unwired: 1 in, 1 out]
            n18 = property on="New Item" class="Bool"(error in=w59, "DisabledEnum"=w60) -> (error out=w62:errorcluster)  [unwired: 1 in, 1 out]
            n19 = property on="Edit Item" class="Bool"(error in=w59, "DisabledEnum"=w60) -> (error out=w63:errorcluster)  [unwired: 1 in, 1 out]
            n20 = property on="Send Follow Up" class="Bool"(error in=w59, "DisabledEnum"=w60) -> (error out=w64:errorcluster)  [unwired: 1 in, 1 out]
            n21 = property on="Delete Item" class="Bool"(error in=w59, "DisabledEnum"=w60) -> (error out=w65:errorcluster)  [unwired: 1 in, 1 out]
            n22 = Merge Errors(w61, w62, w63, w64, w65) -> (w66:errorcluster)
            n23 = flat-sequence {
              tunnel: w66 -> [w97]
              tunnel: [w97] -> w52
              frame #0 {
                n24 = local write "statuBar"("Tables initialization....." ("title")) -> ()
              }
            }
            n25 = Unbundle By Name(w56) -> ("k4b2"=→"k4b2":string[][], "fitmate"=→"fitmate":string[][], "RMR"=→"RMR":string[][], "CPET"=→"CPET":string[][], "BP"=→"BP":string[][], "PP"=→"PP":string[][], "k5"=→"K5":string[][], "bb-pft"=→"BB-PFT":string[][])
            n26 = control-ref of="BB-PFT"() -> (w46:refnum<vi>)
            n27 = control-ref of="K5"() -> (w49:refnum<vi>)
            n28 = control-ref of="RMR"() -> (w87:refnum<vi>)
            n29 = control-ref of="k4b2"() -> (w89:refnum<vi>)
            n30 = control-ref of="CPET"() -> (w86:refnum<vi>)
            n31 = control-ref of="BP"() -> (w85:refnum<vi>)
            n32 = control-ref of="PP"() -> (w84:refnum<vi>)
            n33 = control-ref of="fitmate"() -> (w88:refnum<vi>)
            n34 = call "tableCleaner.vi"("error in (no error)"=w52, "K4b2orK5?"=FALSE, "Table in"=w46, "reference in"=w47) -> ("error out"=w50:errorcluster)  [unwired: 6 in, 1 out]
            n35 = call "tableCleaner.vi"("error in (no error)"=w52, "K4b2orK5?"=TRUE, "Table in"=w49, "reference in"=w47) -> ("error out"=w51:errorcluster)  [unwired: 6 in, 1 out]
            n36 = call "tableCleaner.vi"("error in (no error)"=w52, "K4b2orK5?"=FALSE ("K4b2?"), "Table in"=w87, "reference in"=w47) -> ("error out"=w77:errorcluster)  [unwired: 6 in, 1 out]
            n37 = call "tableCleaner.vi"("error in (no error)"=w52, "K4b2orK5?"=FALSE ("K4b2?"), "Table in"=w86, "reference in"=w47) -> ("error out"=w76:errorcluster)  [unwired: 6 in, 1 out]
            n38 = call "tableCleaner.vi"("error in (no error)"=w52, "K4b2orK5?"=FALSE ("K4b2?"), "Table in"=w85, "reference in"=w47) -> ("error out"=w75:errorcluster)  [unwired: 6 in, 1 out]
            n39 = call "tableCleaner.vi"("error in (no error)"=w52, "K4b2orK5?"=FALSE ("K4b2?"), "Table in"=w84, "reference in"=w47) -> ("error out"=w74:errorcluster)  [unwired: 6 in, 1 out]
            n40 = call "tableCleaner.vi"("error in (no error)"=w52, "K4b2orK5?"=FALSE ("K4b2?"), "Table in"=w88, "reference in"=w47) -> ("error out"=w73:errorcluster)  [unwired: 6 in, 1 out]
            n41 = call "tableCleaner.vi"("error in (no error)"=w52, "K4b2orK5?"=TRUE ("K4b2?"), "Table in"=w89, "reference in"=w47) -> ("error out"=w72:errorcluster)  [unwired: 6 in, 1 out]
            n42 = Merge Errors(w50, w51, w77, w76, w75, w74, w73, w72) -> (w44:errorcluster)
            "title" <- "Cosmed Asia Pacific - Products in Aussie" ("title")
          }
          frame "waitEvent" {
            n43 = event shown="[2] \"New Item\": Mouse Up" {
              selector: _ -> [_ _ _ _ _ _ _ _ _]
              dyn-events: _ -> [_ _ _ _ _ _ _ _ _]
              timeout: 200 -> [_ _ _ _ _ _ _ _ _]
              tunnel: w111 -> [w122 w148 w173 w179 w193 w198 w203 w210 w215]
              tunnel: [w122 w148 w173 w179 w193 w198 w203 w210 w215] -> w104
              tunnel: [state."waitEvent" ("state") state."waitEvent" ("state") state."newItem" ("state") state."searchItem" ("state") w181 state."stop" ("state") state."editItem" ("state") state."sendFollowUp" ("state") state."deleteItem" ("state")] -> w109
              tunnel: [w120 w136 w172 w178 w192 w197 w204 w209 w216] -> w106
              tunnel: w107 -> [w115 _ w170 w176 w190 _ w201 w207 w213]
              tunnel: [w117 w137 w172 w178 w192 w197 w204 w209 w216] -> w105
              tunnel: w103 -> [w116 _ w171 w177 w191 w195 w202 w208 w214]
              tunnel: [w115 w138 w170 w176 w190 "" w201 w207 w213] -> w101
              tunnel: [w116 w142 w171 w177 w191 w195 w202 w208 w214] -> w100
              tunnel: [w113 w135 T4."Disabled and Grayed Out" ("Disabled") T4."Disabled and Grayed Out" ("Disabled") T4."Disabled and Grayed Out" ("Disabled") T4."Disabled and Grayed Out" ("Disabled") T4."Disabled and Grayed Out" ("Disabled") T4."Disabled and Grayed Out" ("Disabled") T4."Disabled and Grayed Out" ("Disabled")] -> w99
              event Timeout {
                n44 = event-data() -> ()  [unwired: 1 in, 2 out]
                n45 = local read "tables"() -> (w114:T1)
                n46 = case shown="\"Pea Pod\"" w114 {
                  tunnel: [T4."Enabled" ("Disabled") T4."Enabled" ("Disabled") T4."Disabled and Grayed Out" ("Disabled") T4."Disabled and Grayed Out" ("Disabled") T4."Disabled and Grayed Out" ("Disabled") T4."Disabled and Grayed Out" ("Disabled") T4."Disabled and Grayed Out" ("Disabled") T4."Disabled and Grayed Out" ("Disabled")] -> w113
                  frame "K4b2", Default {
                  }
                  frame "Fitmate" {
                  }
                  frame "RMR" {
                  }
                  frame "CPET" {
                  }
                  frame "Bod Pod" {
                  }
                  frame "Pea Pod" {
                  }
                  frame "Body Box - PFT" {
                  }
                  frame "K5" {
                  }
                }
                n47 = Equal?(x=w115, y="") -> (x = y?=w119:bool)
                n48 = case shown="False" w119 {
                  tunnel: [T4."Enabled" ("Disabled") T4."Disabled and Grayed Out" ("Disabled")] -> w120
                  tunnel: [T4."Enabled" ("Disabled") T4."Enabled" ("Disabled")] -> w117
                  frame False {
                  }
                  frame True {
                  }
                }
              }
              event Mouse Up {
                n49 = event-data() -> ()  [unwired: 1 in, 7 out]
                n50 = case shown="\"K5\"" "tables" {
                  tunnel: [w154 w156 w158 w160 w162 w164 w165 w167] -> w142
                  tunnel: [T4."Enabled" ("Disabled") T4."Enabled" ("Disabled") T4."Disabled and Grayed Out" ("Disabled") T4."Disabled and Grayed Out" ("Disabled") T4."Disabled and Grayed Out" ("Disabled") T4."Disabled and Grayed Out" ("Disabled") T4."Disabled and Grayed Out" ("Disabled") T4."Disabled and Grayed Out" ("Disabled")] -> w135
                  frame "K4b2", Default {
                    n51 = control-ref of="k4b2"() -> (w154:refnum<vi>)
                  }
                  frame "Fitmate" {
                    n52 = control-ref of="fitmate"() -> (w156:refnum<vi>)
                  }
                  frame "RMR" {
                    n53 = control-ref of="RMR"() -> (w158:refnum<vi>)
                  }
                  frame "CPET" {
                    n54 = control-ref of="CPET"() -> (w160:refnum<vi>)
                  }
                  frame "Bod Pod" {
                    n55 = control-ref of="BP"() -> (w162:refnum<vi>)
                  }
                  frame "Pea Pod" {
                    n56 = control-ref of="PP"() -> (w164:refnum<vi>)
                  }
                  frame "Body Box - PFT" {
                    n57 = control-ref of="BB-PFT"() -> (w165:refnum<vi>)
                  }
                  frame "K5" {
                    n58 = control-ref of="K5"() -> (w167:refnum<vi>)
                  }
                }
                n59 = property on="Property Node" class="Tbl (strict)"(reference=w142) -> ("Value"=w146:string[][], "EditPos"=w147:T6)  [unwired: 1 in, 2 out]
                n60 = Unbundle By Name(w147) -> ("Row"=w144:i32)
                n61 = Index Array(array=w146, index (row)=w144, index (col)=0 ("disabled index (col)")) -> (element=w138:string)
                n62 = Equal?(x=w138, y="") -> (x = y?=w140:bool)
                n63 = case shown="False" w140 {
                  tunnel: [T4."Enabled" ("Disabled") T4."Disabled and Grayed Out" ("Disabled")] -> w136
                  tunnel: [T4."Enabled" ("Disabled") T4."Enabled" ("Disabled")] -> w137
                  frame False {
                  }
                  frame True {
                  }
                }
              }
              event "New Item": Mouse Up {
                w172 = T4."Disabled and Grayed Out" ("Disabled")
                n64 = event-data() -> ()  [unwired: 1 in, 7 out]
              }
              event "Search Item": Mouse Up {
                w178 = T4."Disabled and Grayed Out" ("Disabled")
                n65 = event-data() -> ()  [unwired: 1 in, 7 out]
              }
              event Key Down? {
                w192 = T4."Disabled and Grayed Out" ("Disabled")
                n66 = event-data() -> ("Char"=w184:i16)  [unwired: 1 in, 9 out]
                n67 = To Unsigned Byte Integer(number=w184) -> (unsigned 8bit integer=w188:u8)
                n68 = Type Cast(x=w188) -> (*(type *) &x=w187:string)  [unwired: 1 in]
                n69 = Equal?(x=w187, y="f") -> (x = y?=w185:bool)
                n70 = Select(t=state."searchItem" ("state"), s=w185, f=state."waitEvent" ("state")) -> (s? t:f=w181:T2)
                n71 = event-data() -> ()  [unwired: 2 in, 1 out]
              }
              event "Stop Button": Mouse Up {
                w197 = T4."Disabled and Grayed Out" ("Disabled")
                n72 = event-data() -> ()  [unwired: 1 in, 7 out]
              }
              event "Edit Item": Mouse Up {
                w204 = T4."Disabled and Grayed Out" ("Disabled")
                n73 = event-data() -> ()  [unwired: 1 in, 7 out]
              }
              event "Send Follow Up": Mouse Up {
                w209 = T4."Disabled and Grayed Out" ("Disabled")
                n74 = event-data() -> ()  [unwired: 1 in, 7 out]
              }
              event "Delete Item": Mouse Up {
                w216 = T4."Disabled and Grayed Out" ("Disabled")
                n75 = event-data() -> ()  [unwired: 1 in, 7 out]
              }
            }
            n76 = property on="Send Follow Up" class="Bool"(error in=w104, "DisabledEnum"=w99) -> ()  [unwired: 1 in, 2 out]
            n77 = property on="Delete Item" class="Bool"(error in=w104, "DisabledEnum"=w106) -> ()  [unwired: 1 in, 2 out]
            n78 = property on="Edit Item" class="Bool"(error in=w104, "DisabledEnum"=w106) -> (error out=w102:errorcluster)  [unwired: 1 in, 1 out]
            n79 = property on="Search Item" class="Bool"(error in=w104, "DisabledEnum"=w105) -> ()  [unwired: 1 in, 2 out]
            n80 = property on="New Item" class="Bool"(error in=w104, "DisabledEnum"=w105) -> ()  [unwired: 1 in, 2 out]
          }
          frame "newItem" {
            n81 = property class="Tbl (strict)"(reference=w232, error in=w231) -> (error out=w228:errorcluster, "Label.Text"=w230:string)  [unwired: 1 out]
            n82 = case shown="\"K5\"" w230 {
              tunnel: [deviceType."rmr" ("deviceType") deviceType."bodyBoxPft" ("deviceType") deviceType."fitmate" ("deviceType") deviceType."bp" ("deviceType") deviceType."pp" ("deviceType") deviceType."cpet" ("deviceType") deviceType."k4b2" ("deviceType") deviceType."k5" ("deviceType")] -> w219
              frame "RMR", Default {
              }
              frame "BB-PFT" {
              }
              frame "fitmate" {
              }
              frame "BP" {
              }
              frame "PP" {
              }
              frame "CPET" {
              }
              frame "k4b2" {
              }
              frame "K5" {
              }
            }
            n83 = case shown="True" w218 {
              tunnel: w229 -> [w240 w245]
              tunnel: w228 -> [w239 w243]
              tunnel: [w238 w242] -> w227
              tunnel: [w237 w241] -> w221
              tunnel: w219 -> [w236 w244]
              frame False {
                n84 = call "newDevice.vi"("error in (no error)"=w239, "Device Type"=w236, "reference in"=w240) -> ("error out"=w238:errorcluster, "saved?"=w237:bool)  [unwired: 6 in, 1 out]
              }
              frame True {
                n85 = call "newDeviceLow.vi"("error in (no error)"=w243, "Device Type"=w244, "reference in"=w245) -> ("error out"=w242:errorcluster, "saved?"=w241:bool)  [unwired: 6 in, 1 out]
              }
            }
            n86 = Select(t=TRUE ("saved?"), s=w220, f=w221) -> (s? t:f=w223:bool)
            n87 = Select(t=state."initiate" ("state"), s=w221, f=state."waitEvent" ("state")) -> (s? t:f=w224:T2)
          }
          frame "searchItem" {
            n88 = call "searchEditDevice.vi"("error in (no error)"=w262, "reference in"=w263) -> ("error out"=w261:errorcluster, "saved?"=w255:bool)  [unwired: 7 in, 1 out]
            n89 = Select(t=TRUE ("saved?"), s=w254, f=w255) -> (s? t:f=w256:bool)
            n90 = Select(t=state."initiate" ("state"), s=w255, f=state."waitEvent" ("state")) -> (s? t:f=w258:T2)
          }
          frame "editItem" {
            n91 = property class="Tbl (strict)"(reference=w288, error in=w291) -> (error out=w290:errorcluster, "Label.Text"=w292:string)  [unwired: 1 out]
            n92 = case shown="\"PP\"" w292 {
              tunnel: [deviceType."rmr" ("deviceType") deviceType."k5" ("deviceType") deviceType."bodyBoxPft" ("deviceType") deviceType."fitmate" ("deviceType") deviceType."bp" ("deviceType") deviceType."pp" ("deviceType") deviceType."cpet" ("deviceType") deviceType."k4b2" ("deviceType")] -> w289
              frame "RMR", Default {
              }
              frame "K5" {
              }
              frame "BB-PFT" {
              }
              frame "fitmate" {
              }
              frame "BP" {
              }
              frame "PP" {
              }
              frame "CPET" {
              }
              frame "k4b2" {
              }
            }
            n93 = case shown="True" w268 {
              tunnel: w293 -> [w301 w305]
              tunnel: w290 -> [w300 w302]
              tunnel: w289 -> [w299 w307]
              tunnel: w284 -> [w298 w306]
              tunnel: [w297 w303] -> w277
              tunnel: [w296 w304] -> w270
              frame False {
                n94 = call "editDevice.vi"("error in (no error)"=w300, "S/N IN"=w298, "Device Type In"=w299, "reference in"=w301) -> ("error out"=w297:errorcluster, "saved?"=w296:bool)  [unwired: 5 in, 1 out]
              }
              frame True {
                n95 = call "editDeviceLow.vi"("error in (no error)"=w302, "S/N IN"=w306, "Device Type In"=w307, "reference in"=w305) -> ("error out"=w303:errorcluster, "saved?"=w304:bool)  [unwired: 5 in, 1 out]
              }
            }
            n96 = property on="Property Node" class="Tbl (strict)"(reference=w288, error in=w277) -> (reference out=w283:refnum<vi>, error out=w278:errorcluster, "Value"=w287:string[][])
            n97 = Index Array(array=w287, index (col)=0 ("disabled index (col)")) -> (element=w285:string[])  [unwired: 1 in]
            n98 = Search 1D Array(1D array=w285, element=w284) -> (index of element=w280:i32)  [unwired: 1 in]
            n99 = Bundle By Name(cluster=T6 {"Row"=0, "Column"=0} ("Active Cell:Active Cell"), "Row"=w280, "Column"=0) -> (w281:T6)
            n100 = property on="Property Node" class="Tbl (strict)"(reference=w283, error in=w278, "Index Values"=w281) -> (error out=w276:errorcluster)  [unwired: 1 out]
            n101 = Select(t=TRUE ("saved?"), s=w269, f=w270) -> (s? t:f=w271:bool)
            n102 = Select(t=state."initiate" ("state"), s=w270, f=state."waitEvent" ("state")) -> (s? t:f=w275:T2)
          }
          frame "sendFollowUp" {
            n103 = property class="Tbl (strict)"(reference=w325, error in=w326) -> (error out=w324:errorcluster, "Label.Text"=w317:string)  [unwired: 1 out]
            n104 = case shown="\"K5\"" w317 {
              tunnel: [deviceType."rmr" ("deviceType") deviceType."k5" ("deviceType") deviceType."bodyBoxPft" ("deviceType") deviceType."fitmate" ("deviceType") deviceType."bodyBoxPft" ("deviceType") deviceType."bp" ("deviceType") deviceType."cpet" ("deviceType") deviceType."k4b2" ("deviceType")] -> w316
              frame "RMR", Default {
              }
              frame "K5" {
              }
              frame "BB-PFT" {
              }
              frame "fitmate" {
              }
              frame "BP" {
              }
              frame "PP" {
              }
              frame "CPET" {
              }
              frame "k4b2" {
              }
            }
            n105 = call "followUpDevice.vi"("error in (no error)"=w324, "S/N"=w322, "Device Type"=w316, "reference in"=w323) -> ("error out"=w319:errorcluster)  [unwired: 6 in, 1 out]
            n106 = case shown="No Error" w319 {
              selector: w319 -> [w337 w350]
              tunnel: [w338 state."waitEvent" ("state")] -> w321
              tunnel: [w337 w348] -> w318
              frame No Error {
                n107 = flat-sequence {
                  tunnel: [w341] -> w338
                  frame #0 {
                    n108 = Two Button Dialog(message="Do you want to update the Follow Up sent Date?", 1:"No" ("F button name (\"Cancel\")"), 2:"Yes" ("T button name (\"OK\")")) -> (T button?=w340:bool)
                    n109 = Select(t=state."editItem", s=w340, f=state."waitEvent" ("state")) -> (s? t:f=w341:T2)
                  }
                }
              }
              frame Error {
                n110 = call <vilib>:"Simple Error Handler.vi"("error in (no error)"=w350) -> ("source out"=w346:string, "error out"=w349:errorcluster)  [unwired: 4 in, 3 out]
                n111 = call <vilib>:"Clear Errors.vi"("error in (no error)"=w349) -> ("error out"=w348:errorcluster)  [unwired: 5 in, 1 out]
                n112 = One Button Dialog(message=w346, button name ("OK")="OK" ("T button name (\"OK\")")) -> ()  [unwired: 1 out]
              }
            }
          }
          frame "deleteItem" {
            n113 = property class="Tbl (strict)"(reference=w363, error in=w365) -> (error out=w364:errorcluster, "Label.Text"=w354:string)  [unwired: 1 out]
            n114 = case shown="\"K5\"" w354 {
              tunnel: [deviceType."rmr" ("deviceType") deviceType."k5" ("deviceType") deviceType."bodyBoxPft" ("deviceType") deviceType."fitmate" ("deviceType") deviceType."bodyBoxPft" ("deviceType") deviceType."bp" ("deviceType") deviceType."cpet" ("deviceType") deviceType."k4b2" ("deviceType")] -> w353
              frame "RMR", Default {
              }
              frame "K5" {
              }
              frame "BB-PFT" {
              }
              frame "fitmate" {
              }
              frame "BP" {
              }
              frame "PP" {
              }
              frame "CPET" {
              }
              frame "k4b2" {
              }
            }
            n115 = case shown="True" w352 {
              tunnel: [w375 w377] -> w367
              tunnel: w366 -> [w374 w381]
              tunnel: w364 -> [w373 w378]
              tunnel: w362 -> [w372 w379]
              tunnel: [w371 w376] -> w356
              tunnel: w353 -> [w370 w380]
              frame False {
                n116 = call "deleteDevice.vi"("error in (no error)"=w373, "S/N IN"=w372, "Device Type In"=w370, "reference in"=w374) -> ("error out"=w375:errorcluster, "saved?"=w371:bool)  [unwired: 5 in, 1 out]
              }
              frame True {
                n117 = call "deleteDeviceLow.vi"("error in (no error)"=w378, "S/N IN"=w379, "Device Type In"=w380, "reference in"=w381) -> ("error out"=w377:errorcluster, "saved?"=w376:bool)  [unwired: 5 in, 1 out]
              }
            }
            n118 = Select(t=TRUE ("saved?"), s=w355, f=w356) -> (s? t:f=w357:bool)
            n119 = Select(t=state."initiate" ("state"), s=w356, f=state."waitEvent" ("state")) -> (s? t:f=w359:T2)
          }
          frame "stop" {
            n120 = case shown="True" w391 {
              tunnel: w393 -> [w404 w407]
              tunnel: [w404 w408] -> w392
              tunnel: w390 -> [_ w405]
              frame False {
              }
              frame True {
                n121 = flat-sequence {
                  tunnel: w407 -> [w409]
                  tunnel: [w409] -> w406
                  frame #0 {
                    n122 = local write "statuBar"("Wait....I'm saving the new data on the excel file" ("statuBar")) -> ()
                  }
                }
                n123 = call "saveData.vi"("error in (no error)"=w406, "reference in"=w405) -> ("error out"=w408:errorcluster)  [unwired: 8 in, 1 out]
              }
            }
            n124 = Unbundle By Name(w392) -> ("status"=w396:bool)
            n125 = Not(x=w396) -> (.not. x?=w395:bool)
            n126 = case shown="True" w396 {
              tunnel: w392 -> [_ w412]
              frame False {
              }
              frame True {
                n127 = Unbundle By Name(w412) -> ("source"=w411:string)
                n128 = Concatenate Strings("An Error occur: " ("message"), w411) -> (w414:string)
                n129 = One Button Dialog(message=w414) -> ()  [unwired: 1 in, 1 out]
              }
            }
            n130 = Select(t="Stoped from User" ("title"), s=w395, f="Stoped for an Error" ("title")) -> (s? t:f=w398:string)
          }
        }
        "statuBar" <- w30
        "Item Selected (S/N):" <- w29
        n131 = Unbundle By Name(w37) -> ("status"=w36:bool)
        n132 = Not(x=w36) -> (.not. x?=w33:bool)
        n133 = Select(t=w35, s=w33, f=state."stop") -> (s? t:f=w34:T2)
      }
    }
    frame Error {
    }
  }
  "error out" <- w3
  "reference out" <- w1
